vi "ASI_Ask_position.vi"(8 "error in":errorcluster, 10 "Axis":u16(ring)=2 items=["X", "Y", "Z"], 11 "VISA resource name":refnum<visa-resource-name>) -> (0 "error out":errorcluster, 2 "Current Z position (um)":dbl, 3 "VISA resource name out":refnum<visa-resource-name>)   [LabVIEW 2018]
panel:
  out "Serial Settings:Number of Bytes at Serial Port":u32
  out "read buffer":string
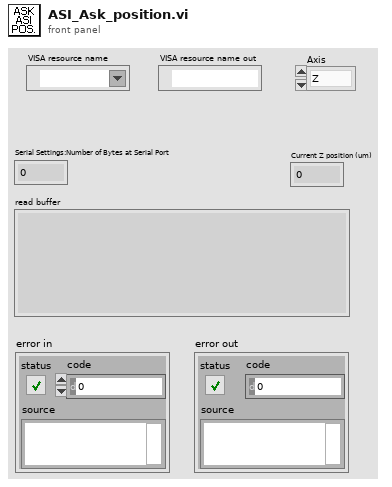
[diagram p1: front panel]
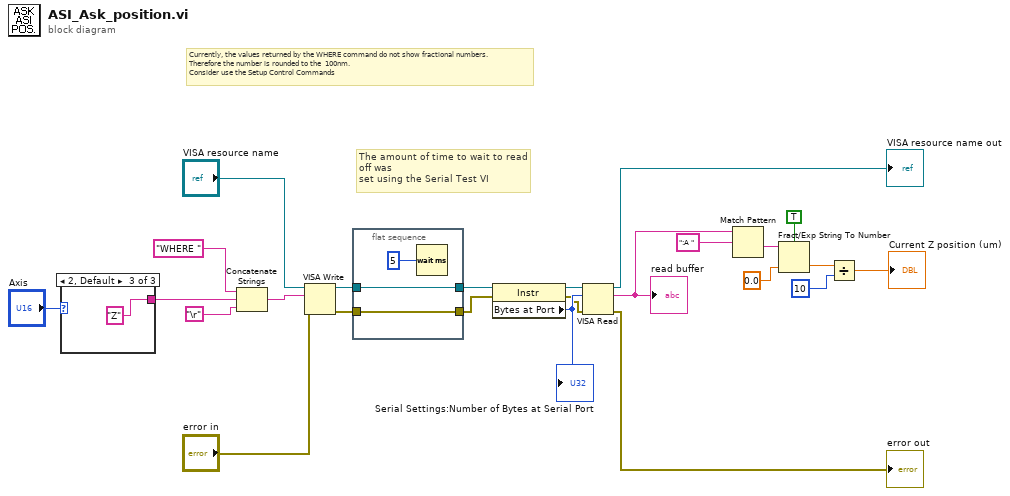
[diagram p0: block diagram]
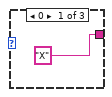
[diagram p2: hidden frame]
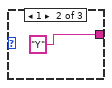
[diagram p3: hidden frame]
diagram:
  # "Currently, the values returned by the WHERE command do not show fractional numbers.\nTherefore the number is rounded to the  100nm. \nConsider use the Setup Control Commands"
  # "The amount of time to wait to read off was \nset using the Serial Test VI"
  n1 = case shown="2, Default" "Axis" {
    tunnel: ["X" "Y" "Z"] -> w1
    frame 0 {
    }
    frame 1 {
    }
    frame 2, Default {
    }
  }
  n2 = Concatenate Strings("WHERE " ("string"), w1, "\r") -> (w7:string)
  n3 = VISA Write(VISA resource name="VISA resource name", write buffer=w7, error in (no error)="error in") -> (VISA resource name out=w21:refnum<visa-resource-name>, error out=w17:errorcluster)  [unwired: 1 out]
  n4 = flat-sequence {
    tunnel: [w30] -> w22
    tunnel: w21 -> [w30]
    tunnel: [w28] -> w18
    tunnel: w17 -> [w28]
    frame #0 {
      n5 = Wait (ms)(milliseconds to wait=u32 5) -> ()  [unwired: 1 out]
    }
  }
  n6 = property class="Instr"(reference=w22, error in=w18) -> (reference out=w24:refnum<visa-resource-name>, error out=w16:errorcluster, "Bytes at Port"=w23:u32)
  "Serial Settings:Number of Bytes at Serial Port" <- w23
  n7 = VISA Read(VISA resource name=w24, byte count=w23, error in (no error)=w16) -> (VISA resource name out=→"VISA resource name out":refnum<visa-resource-name>, read buffer=w13:string, error out=→"error out":errorcluster)  [unwired: 1 out]
  "read buffer" <- w13
  n8 = Match Pattern(string=w13, regular expression=":A " ("search string/char (-)")) -> (after substring=w11:string)  [unwired: 1 in, 3 out]
  n9 = Fract/Exp String To Number(use system decimal point (T)=TRUE, string=w11, default (0 dbl)=0.0 ("default (0 I32)")) -> (number=w10:dbl)  [unwired: 1 in, 1 out]
  n10 = Divide(x=w10, y=10) -> (x/y=→"Current Z position (um)":dbl)
